vi "Practica4_WhileLoop.vi"() -> ()   [LabVIEW 2022 SP3]
panel:
  out "Si se encontró\nNo se encontró":bool
  out "CantidadEjecuciones":dbl
  out "ValorGenerado":dbl
  in  "ValorBuscado":dbl
  # "Anahí Montserrat Vázquez Padilla \nPráctica 04: While loop \n06/02/2024"
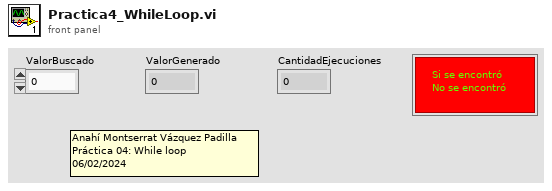
[diagram p1: front panel]
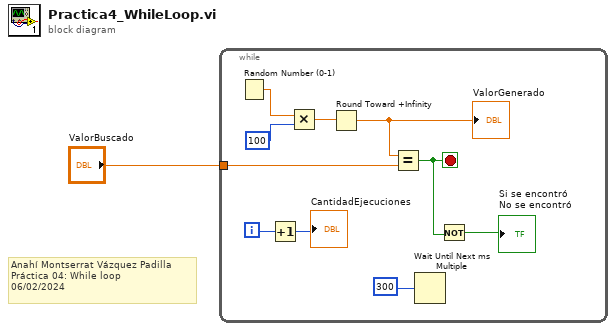
[diagram p0: block diagram]
diagram:
  # "Anahí Montserrat Vázquez Padilla \nPráctica 04: While loop \n06/02/2024"
  n1 = while {
    tunnel: "ValorBuscado" -> [w7]
    i -> [w5]
    stop <- w3 stop-if-true
    n2 = Random Number (0-1)() -> (number: 0 to 1=w10:dbl)
    n3 = Increment(x=w5) -> (x+1=→"CantidadEjecuciones":i32)
    n4 = Multiply(x=w10, y=100) -> (x*y=w9:dbl)
    n5 = Round Toward +Infinity(x=w9) -> (ceil(x): smallest int >= x=w8:dbl)
    "ValorGenerado" <- w8
    n6 = Equal?(x=w8, y=w7) -> (x = y?=w3:bool)
    n7 = Wait Until Next ms Multiple(millisecond multiple=300) -> ()  [unwired: 1 out]
    n8 = Not(x=w3) -> (.not. x?=→"Si se encontró\nNo se encontró":bool)
  }
